vi "Array to Array of VData.vi"(8 "错误输入":errorcluster, 10 "MultiD Array":variant) -> (0 "错误输出":errorcluster, 2 "1D Array of Variants":variant[](array[variant]))   [LabVIEW 2012, in "TD Tools.lvlib"]
uses:
  TD Tools.lvlib
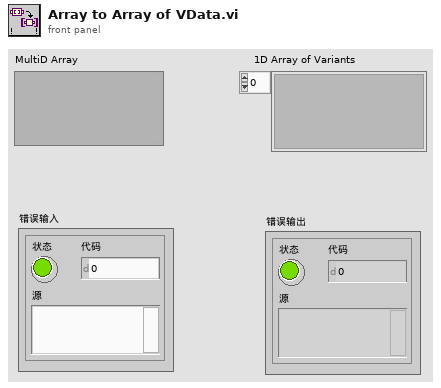
[diagram p1: front panel]
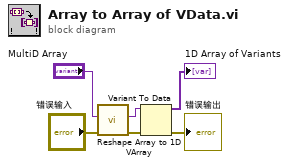
[diagram p0: block diagram]
diagram:
  n1 = call "Reshape Array to 1D VArray.vi"("error in (no error)"="错误输入", "MultiD Array"="MultiD Array") -> ("error out"=w2:errorcluster, "1D VArray"=w4:variant)  [unwired: 7 in, 1 out]
  n2 = Variant To Data(error in=w2, Variant=w4) -> (data=→"1D Array of Variants":variant[], error out=→"错误输出":errorcluster)  [unwired: 1 in]
